vi "Global-Led.vi"() -> ()   [LabVIEW 2020]
panel:
  in  "LED-control states fr":T1(ring)
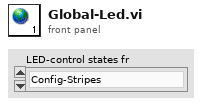
[diagram p1: front panel]
types:
  T1 = enum16{"Config-Stripes", "swapperlines", "Rand", "Solid", "Flash-S", "Gradyent", "Move-Stripes", "Org-Rand", "Move-Point-Tail", "Flames", "Alt-Colors"}
diagram:
